vi "Assign 3 Stair Case Light (1).vi"() -> ()   [LabVIEW 2021]
panel:
  in  "?":string
  out "Y=A'B+A'B":bool
  in  "Ground Floor Switch A":bool
  in  "First Floor Switch B":bool
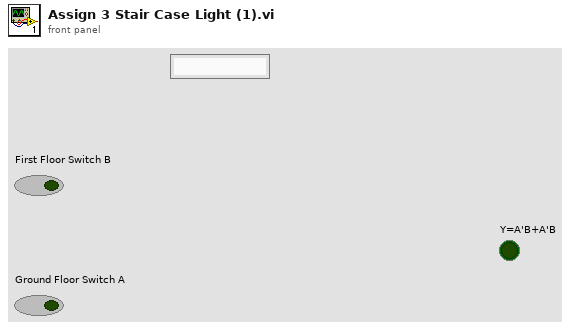
[diagram p1: front panel]
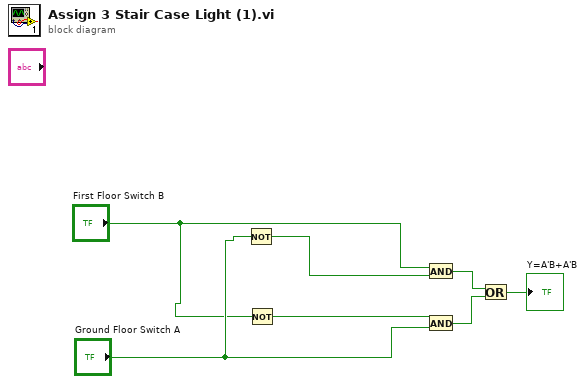
[diagram p0: block diagram]
diagram:
  n1 = Not(x="Ground Floor Switch A") -> (.not. x?=w3:bool)
  n2 = Not(x="First Floor Switch B") -> (.not. x?=w1:bool)
  n3 = And(x="First Floor Switch B", y=w3) -> (x .and. y?=w5:bool)
  n4 = And(x=w1, y="Ground Floor Switch A") -> (x .and. y?=w6:bool)
  n5 = Or(x=w5, y=w6) -> (x .or. y?=→"Y=A'B+A'B":bool)
